vi "String to Datatype.vi"(11 "String Value":string) -> (3 "Prop.DataType":i32)   [LabVIEW 2015, in "SLSC Remote.lvclass"]
uses:
  SLSC Remote.lvclass
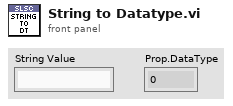
[diagram p1: front panel]
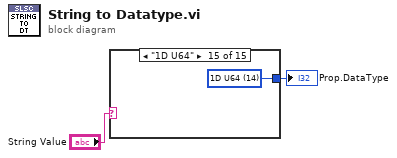
[diagram p0: block diagram]
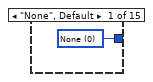
[diagram p2: hidden frame]
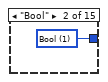
[diagram p3: hidden frame]
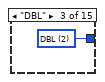
[diagram p4: hidden frame]
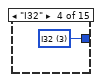
[diagram p5: hidden frame]
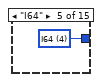
[diagram p6: hidden frame]
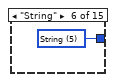
[diagram p7: hidden frame]
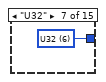
[diagram p8: hidden frame]
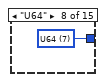
[diagram p9: hidden frame]
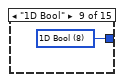
[diagram p10: hidden frame]
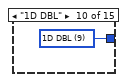
[diagram p11: hidden frame]
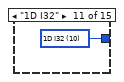
[diagram p12: hidden frame]
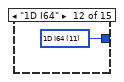
[diagram p13: hidden frame]
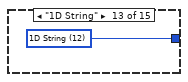
[diagram p14: hidden frame]
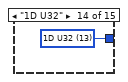
[diagram p15: hidden frame]
diagram:
  n1 = case shown="\"1D U64\"" "String Value" {
    tunnel: [w3 w4 w5 w6 w7 w8 w9 w10 w11 w12 w13 w14 w15 w16 w17] -> w2
    frame "None", Default {
      w3 = 0 items=["None", "Bool", "DBL", "I32", "I64", "String", "U32", "U64", "1D Bool", "1D DBL", "1D I32", "1D I64", "1D String", "1D U32", "1D U64"] ("Prop.DataType")
    }
    frame "Bool" {
      w4 = 1 items=["None", "Bool", "DBL", "I32", "I64", "String", "U32", "U64", "1D Bool", "1D DBL", "1D I32", "1D I64", "1D String", "1D U32", "1D U64"] ("Prop.DataType")
    }
    frame "DBL" {
      w5 = 2 items=["None", "Bool", "DBL", "I32", "I64", "String", "U32", "U64", "1D Bool", "1D DBL", "1D I32", "1D I64", "1D String", "1D U32", "1D U64"] ("Prop.DataType")
    }
    frame "I32" {
      w6 = 3 items=["None", "Bool", "DBL", "I32", "I64", "String", "U32", "U64", "1D Bool", "1D DBL", "1D I32", "1D I64", "1D String", "1D U32", "1D U64"] ("Prop.DataType")
    }
    frame "I64" {
      w7 = 4 items=["None", "Bool", "DBL", "I32", "I64", "String", "U32", "U64", "1D Bool", "1D DBL", "1D I32", "1D I64", "1D String", "1D U32", "1D U64"] ("Prop.DataType")
    }
    frame "String" {
      w8 = 5 items=["None", "Bool", "DBL", "I32", "I64", "String", "U32", "U64", "1D Bool", "1D DBL", "1D I32", "1D I64", "1D String", "1D U32", "1D U64"] ("Prop.DataType")
    }
    frame "U32" {
      w9 = 6 items=["None", "Bool", "DBL", "I32", "I64", "String", "U32", "U64", "1D Bool", "1D DBL", "1D I32", "1D I64", "1D String", "1D U32", "1D U64"] ("Prop.DataType")
    }
    frame "U64" {
      w10 = 7 items=["None", "Bool", "DBL", "I32", "I64", "String", "U32", "U64", "1D Bool", "1D DBL", "1D I32", "1D I64", "1D String", "1D U32", "1D U64"] ("Prop.DataType")
    }
    frame "1D Bool" {
      w11 = 8 items=["None", "Bool", "DBL", "I32", "I64", "String", "U32", "U64", "1D Bool", "1D DBL", "1D I32", "1D I64", "1D String", "1D U32", "1D U64"] ("Prop.DataType")
    }
    frame "1D DBL" {
      w12 = 9 items=["None", "Bool", "DBL", "I32", "I64", "String", "U32", "U64", "1D Bool", "1D DBL", "1D I32", "1D I64", "1D String", "1D U32", "1D U64"] ("Prop.DataType")
    }
    frame "1D I32" {
      w13 = 10 items=["None", "Bool", "DBL", "I32", "I64", "String", "U32", "U64", "1D Bool", "1D DBL", "1D I32", "1D I64", "1D String", "1D U32", "1D U64"] ("Prop.DataType")
    }
    frame "1D I64" {
      w14 = 11 items=["None", "Bool", "DBL", "I32", "I64", "String", "U32", "U64", "1D Bool", "1D DBL", "1D I32", "1D I64", "1D String", "1D U32", "1D U64"] ("Prop.DataType")
    }
    frame "1D String" {
      w15 = 12 items=["None", "Bool", "DBL", "I32", "I64", "String", "U32", "U64", "1D Bool", "1D DBL", "1D I32", "1D I64", "1D String", "1D U32", "1D U64"] ("Prop.DataType")
    }
    frame "1D U32" {
      w16 = 13 items=["None", "Bool", "DBL", "I32", "I64", "String", "U32", "U64", "1D Bool", "1D DBL", "1D I32", "1D I64", "1D String", "1D U32", "1D U64"] ("Prop.DataType")
    }
    frame "1D U64" {
      w17 = 14 items=["None", "Bool", "DBL", "I32", "I64", "String", "U32", "U64", "1D Bool", "1D DBL", "1D I32", "1D I64", "1D String", "1D U32", "1D U64"] ("Prop.DataType")
    }
  }
  "Prop.DataType" <- w2
